vi "test_COM_2.vi"() -> ()   [LabVIEW 2019]
panel:
  out "return count":u32
  out "error out":errorcluster
  in  "stop":bool
  out "read buffer":string
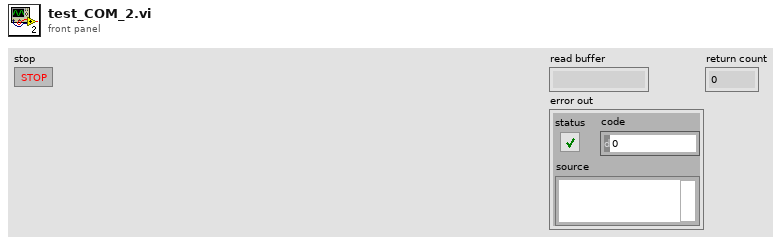
[diagram p1: front panel]
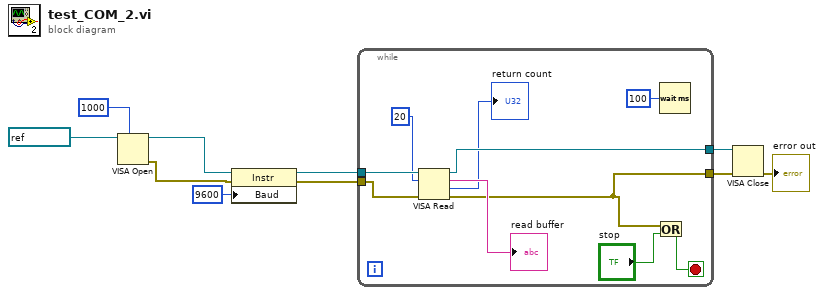
[diagram p0: block diagram]
diagram:
  n1 = VISA Open(timeout (0)=u32 1000 ("VISA Open timeout (0)"), VISA resource name=refnum<visa-resource-name> "COM3") -> (VISA resource name=w10:refnum<visa-resource-name>, error out=w6:errorcluster)  [unwired: 3 in]
  n2 = property class="Instr"(reference=w10, error in=w6, "Baud"=u32 9600 ("Serial Settings:Baud Rate")) -> (reference out=w8:refnum<visa-resource-name>, error out=w7:errorcluster)
  n3 = while {
    tunnel: w8 -> [w20]
    tunnel: w7 -> [w19]
    tunnel: [w18] -> w4
    tunnel: [w14] -> w3
    stop <- w12 stop-if-true
    n4 = VISA Read(VISA resource name=w20, byte count=u32 20, error in (no error)=w19) -> (VISA resource name out=w18:refnum<visa-resource-name>, read buffer=→"read buffer":string, return count=→"return count":u32, error out=w14:errorcluster)
    n5 = Or(x=w14, y="stop") -> (x .or. y?=w12:bool)
    n6 = Wait (ms)(milliseconds to wait=u32 100) -> ()  [unwired: 1 out]
  }
  n7 = VISA Close(VISA resource name=w4, error in (no error)=w3) -> (error out=→"error out":errorcluster)
